vi "Open System Definition.vi"(8 "error in":errorcluster, 11 "system definition file":path) -> (0 "error out":errorcluster, 1 "target":refnum<k24>, 2 "root":refnum<k24>, 3 "system definition":refnum<k24>)   [LabVIEW 2020, in "AIM ARINC 664 Scripting Examples.lvlib"]
uses:
  AIM ARINC 664 Scripting Examples.lvlib
  NationalInstruments.VeriStand.SystemDefinitionAPI
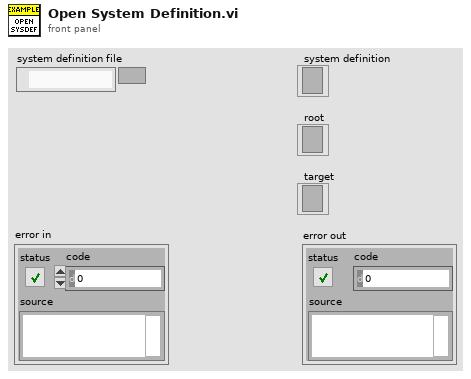
[diagram p1: front panel]
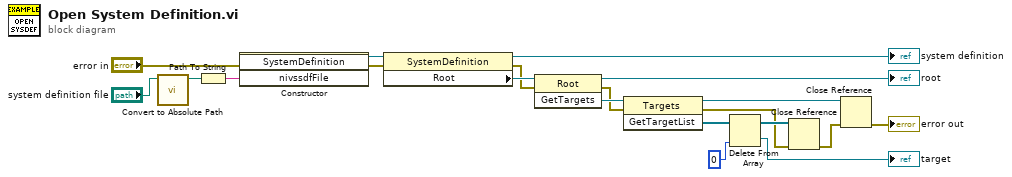
[diagram p0: block diagram]
diagram:
  n1 = call "Convert to Absolute Path.vi"("system definition file"="system definition file") -> ("absolute path"=w1:path)  [unwired: 10 in]
  n2 = Path To String(path=w1) -> (string=w3:string)
  n3 = constructor class="SystemDefinition"(error in="error in", "nivssdfFile"=w3) -> (reference out=w6:refnum<k24>, error out=w5:errorcluster)  [unwired: 2 in, 2 out]
  n4 = property class="SystemDefinition"(reference=w6, error in=w5) -> (reference out=→"system definition":refnum<k24>, error out=w7:errorcluster, "Root"=w8:refnum<k24>)
  n5 = invoke class="Root" method="GetTargets"(reference=w8, error in=w7) -> (reference out=→"root":refnum<k24>, error out=w9:errorcluster, "GetTargets"=w10:refnum<k24>)  [unwired: 1 in]
  n6 = invoke class="Targets" method="GetTargetList"(reference=w10, error in=w9) -> (reference out=w16:refnum<k24>, error out=w13:errorcluster, "GetTargetList"=w11:refnum<k24>[])  [unwired: 1 in]
  n7 = Delete From Array(array=w11, index=0) -> (deleted portion=→"target":refnum<k24>, array with subset deleted=w14:refnum<k24>[])  [unwired: 1 in]
  n8 = Close Reference(reference=w14, error in (no error)=w13) -> (error out=w15:errorcluster)
  n9 = Close Reference(reference=w16, error in (no error)=w15) -> (error out=→"error out":errorcluster)
